vi "Error Handler.vi"(1 "Return Value":i32) -> (0 "error out":errorcluster)   [LabVIEW 2018, in "Laser.lvlib"]
uses:
  <vilib>/ErrorRing/Error Ring.xnode
  Laser.lvlib
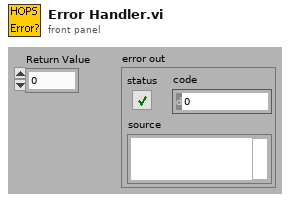
[diagram p1: front panel]
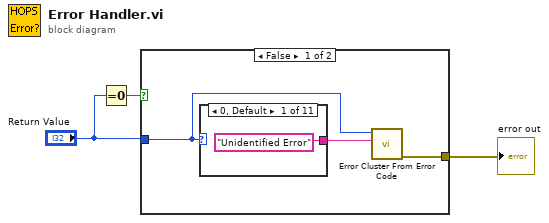
[diagram p0: block diagram]
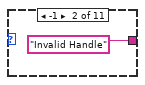
[diagram p2: hidden frame]
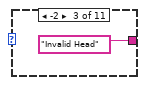
[diagram p3: hidden frame]
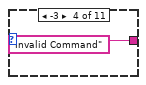
[diagram p4: hidden frame]
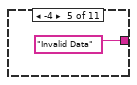
[diagram p5: hidden frame]
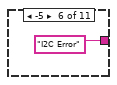
[diagram p6: hidden frame]
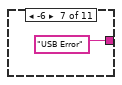
[diagram p7: hidden frame]
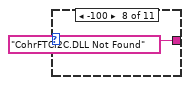
[diagram p8: hidden frame]
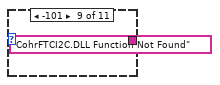
[diagram p9: hidden frame]
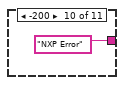
[diagram p10: hidden frame]
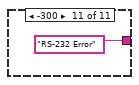
[diagram p11: hidden frame]
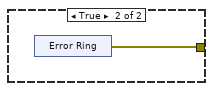
[diagram p12: hidden frame]
diagram:
  n1 = Equal To 0?(x="Return Value") -> (x = 0?=w3:bool)
  n2 = case shown="False" w3 {
    tunnel: "Return Value" -> [w5 _]
    tunnel: [w4 w18] -> w1
    frame False {
      n3 = case shown="0, Default" w5 {
        tunnel: ["Unidentified Error" "Invalid Handle" "Invalid Head" "Invalid Command" "Invalid Data" "I2C Error" "USB Error" "CohrFTCI2C.DLL Not Found" "CohrFTCI2C.DLL Function Not Found" "NXP Error" "RS-232 Error"] -> w6
        frame 0, Default {
        }
        frame -1 {
        }
        frame -2 {
        }
        frame -3 {
        }
        frame -4 {
        }
        frame -5 {
        }
        frame -6 {
        }
        frame -100 {
        }
        frame -101 {
        }
        frame -200 {
        }
        frame -300 {
        }
      }
      n4 = call <vilib>:"Error Cluster From Error Code.vi"("error message (\"\")"=w6, "error code (0)"=w5) -> ("error out"=w4:errorcluster)  [unwired: 7 in]
    }
    frame True {
      n5 = xnode "Error Ring"() -> ("error out"=w18:errorcluster)
    }
  }
  "error out" <- w1
